vi "XML Sandbox.vi"() -> ()   [LabVIEW 2019, in "Control Experiment.lvclass"]
uses:
  Control Experiment.lvclass
  <userlib>/LevyLab/Levylab Instruments/SMOs/Instrument/Instrument.lvclass
  <userlib>/_OpenG.lib/file/file.llb/Compare Two Paths - Scalar__ogtk.vi
panel:
  out "Array":string[](array[string])
  out "Installed Instruments":path[](array[path])
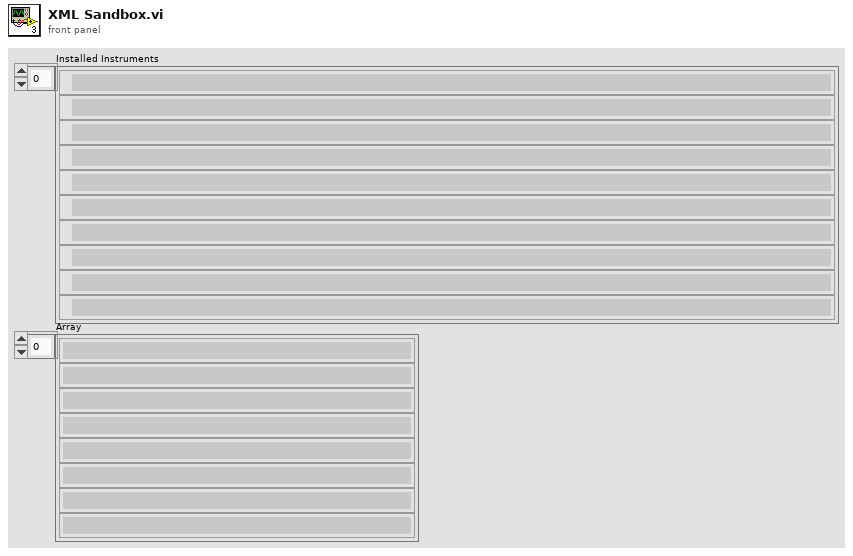
[diagram p1: front panel]
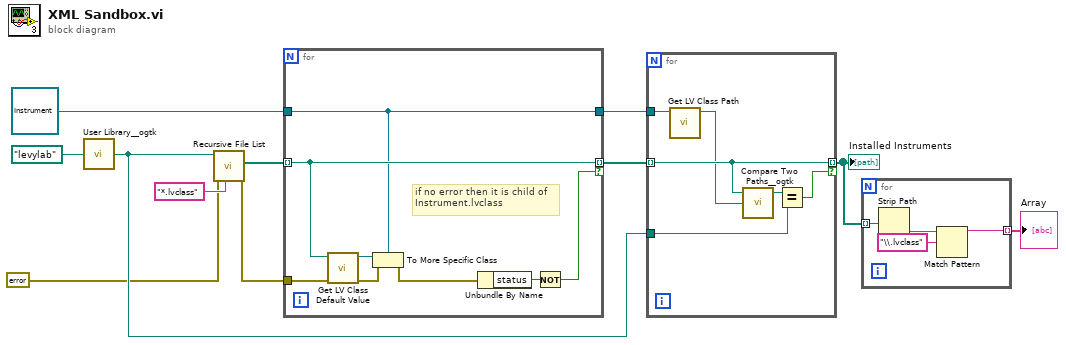
[diagram p0: block diagram]
diagram:
  n1 = call <userlib>:"User Library__ogtk.vi"("Relative path (.)"=path "levylab") -> ("User Library (+ Relative)"=w7:path)
  n2 = call <vilib>:"Recursive File List.vi"("pattern"="*.lvclass", "error in (no error)"=errorcluster {"status"=FALSE, "code"=0, "source"=""}, "Folder Path"=w7) -> ("error out"=w6:errorcluster, "All Files in Dir"=w9:path[])  [unwired: 4 in, 3 out]
  n3 = for {
    tunnel: [w18] -> w8 mode=indexing if=w19
    tunnel: w9 -> [w18] mode=indexing
    tunnel: refnum<class "Instrument.lvclass"> refnum ("Instrument.lvclass") -> [w12]
    tunnel: w6 -> [w13]
    tunnel: [w12] -> w3
    # "if no error then it is child of\nInstrument.lvclass"
    n4 = call <vilib>:"Get LV Class Default Value.vi"("error in (no error)"=w13, "class path"=w18) -> ("error out"=w16:errorcluster, "object"=w17:refnum<class>)  [unwired: 8 in]
    n5 = To More Specific Class(target class=w12, reference=w17, error in=w16) -> (error out=w14:errorcluster)  [unwired: 1 out]
    n6 = Unbundle By Name(w14) -> ("status"=w15:bool)
    n7 = Not(x=w15) -> (.not. x?=w19:bool)
  }
  n8 = for {
    tunnel: w8 -> [w23] mode=indexing
    tunnel: [w23] -> w2 mode=indexing if=w20
    tunnel: w7 -> [w25]
    tunnel: w3 -> [w21]
    n9 = call <vilib>:"Get LV Class Path.vi"("object"=w21) -> ("class path"=w22:path)  [unwired: 9 in, 1 out]
    n10 = call-poly <userlib>:"Compare Two Paths__ogtk.vi"("path2"=w22, "path1"=w23) -> ("common path"=w24:path)  [unwired: 1 in, 2 out]
    n11 = Equal?(x=w24, y=w25) -> (x = y?=w20:bool)
  }
  "Installed Instruments" <- w2
  n12 = for {
    tunnel: w2 -> [w29] mode=indexing
    tunnel: [w26] -> w1 mode=indexing
    n13 = Strip Path(path=w29) -> (name=w28:string)  [unwired: 1 out]
    n14 = Match Pattern(string=w28, regular expression="\\.lvclass") -> (before substring=w26:string)  [unwired: 1 in, 3 out]
  }
  "Array" <- w1
